vi "who_am_i.vi"(8 "error in":errorcluster, 11 "Nominal Client in":refnum<class "Nominal Client.lvclass">) -> (0 "error out":errorcluster, 2 "User":refnum<class "User.lvclass">, 3 "Nominal Client out":refnum<class "Nominal Client.lvclass">)   [LabVIEW 2020, in "Nominal Client.lvclass"]
doc: "Gets the profile of the authenticated user."
uses:
  Nominal Client.lvclass
  Nominal Client.lvclass/Nominal Client.ctl
  create.authorization_header.vi
  trace.payload_sent.vi
  trace.payload_received.vi
  error.vi
  api_token.get.vi
  trace.calling_method.vi
  <vilib>/JDP Science/JDP Science Common Utilities/Trim Whitespace__JDP.vi
  <vilib>/AdvancedString/1D String Array to Delimited String.vi
  error.vi/859f8e04-e495-489b-b5b4-7ac163f56130.vi
  <vilib>/Utility/libraryn.llb/Get File Extension.vi
  log_file.write.vi
  submodules/reqwest-labview/lv-src/reqwest/get.vi
  <vilib>/JDP Science/JSONtext/Get all Object Items.vi
  <vilib>/Utility/error.llb/Error Cluster From Error Code.vi
  <vilib>/JDP Science/JSONtext/JSON text to Variant.vi
  <vilib>/JDP Science/JSONtext/LVClass Serializer/JSONtext LVClass Serializer.lvclass
  User/User.lvclass
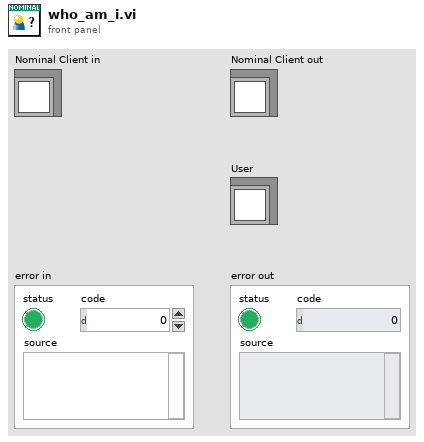
[diagram p1: front panel]
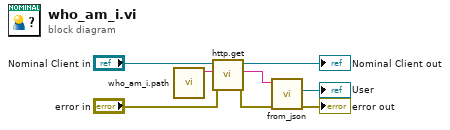
[diagram p0: block diagram]
diagram:
  n1 = call "who_am_i.path.vi"() -> ("path"=w8:string)  [unwired: 11 in]
  n2 = call "http.get.vi"("error in"="error in", "Path"=w8, "Nominal Client in"="Nominal Client in") -> ("error out"=w1:errorcluster, "Response"=w4:string, "Nominal Client out"=→"Nominal Client out":refnum<class "Nominal Client.lvclass">)  [unwired: 6 in]
  n3 = call "from_json.vi"("error in"=w1, "JSON"=w4) -> ("error out"=→"error out":errorcluster, "User"=→"User":refnum<class "User.lvclass">)  [unwired: 8 in]
